vi "GetParam.vi"(8 "error in (no error)":errorcluster caption="entrée d'erreur (pas d'erreur)", 11 "quantile_transform.lvclass":refnum<class "quantile_transform.lvclass">) -> (0 "error out":errorcluster caption="sortie d'erreur", 2 "quantile_transform":T1={"axis"=0, "n_quantiles"=1000, "output_distribution"="uniform", "ignore_implicit_zeros"=FALSE, "subsample"=100000.0, "random_state"=-1, "copy"=TRUE} {"random_state" min=-1}, 3 "quantile_transform.lvclass":refnum<class "quantile_transform.lvclass">)   [LabVIEW 2020, in "quantile_transform.lvclass"]
doc: "Get Parameters"
uses:
  quantile_transform.lvclass
  quantile_transform.lvclass/quantile_transform.ctl
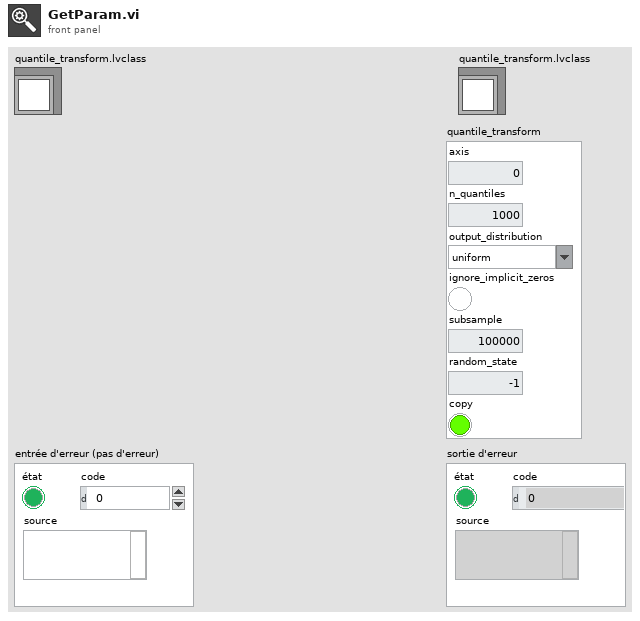
[diagram p1: front panel]
types:
  T1 = cluster{"axis":i32, "n_quantiles":i32, "output_distribution":string, "ignore_implicit_zeros":bool, "subsample":dbl, "random_state":i32, "copy":bool}
  T2 = cluster{"axis":u8, "n_quantiles":i32, "output_distribution":string, "ignore_implicit_zeros":bool, "subsample":dbl, "random_state":i32, "copy":bool}
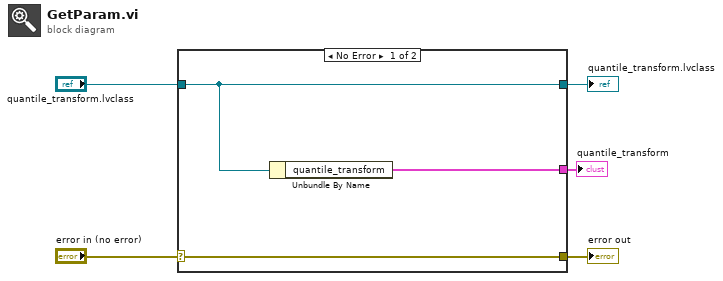
[diagram p0: block diagram]
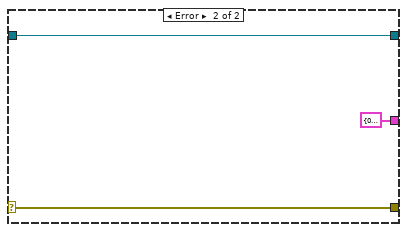
[diagram p2: hidden frame]
diagram:
  n1 = case shown="No Error" "error in (no error)" {
    selector: "error in (no error)" -> [w8 w10]
    tunnel: [w8 w10] -> w4
    tunnel: [w7 w11] -> w2
    tunnel: "quantile_transform.lvclass" -> [w7 w11]
    tunnel: [w6 T2 {"axis"=0, "n_quantiles"=0, "output_distribution"="", "ignore_implicit_zeros"=FALSE, "subsample"=0.0, "random_state"=0, "copy"=FALSE} ("quantile_transform")] -> w1
    frame No Error {
      n2 = Unbundle By Name(w7) -> ("quantile_transform"=w6:T1)
    }
    frame Error {
    }
  }
  "error out" <- w4
  "quantile_transform.lvclass" <- w2
  "quantile_transform" <- w1
